vi "readWatchDog.vi"(8 "error in (no error)":errorcluster, 10 "id":T5=1, 11 "CoolerControler in":refnum<class "CoolerControler.lvclass">) -> (0 "error out":errorcluster, 1 "AS":T2, 2 "PS":T3, 3 "CoolerControler out":refnum<class "CoolerControler.lvclass">, 4 "WS":T1, 5 "CS":T4)   [LabVIEW 2016, in "CoolerControler.lvclass"]
uses:
  CoolerControler.lvclass
  typedefs/CoolerId.ctl
  typedefs/ControlStatusMode.ctl
  typedefs/PumpStatusFlag.ctl
  typedefs/AlarmStatusFlag.ctl
  typedefs/WarningStatusFlag.ctl
  typedefs/CoolerQuery.ctl
  SerialCommand/CoolerSerialCommand.lvclass
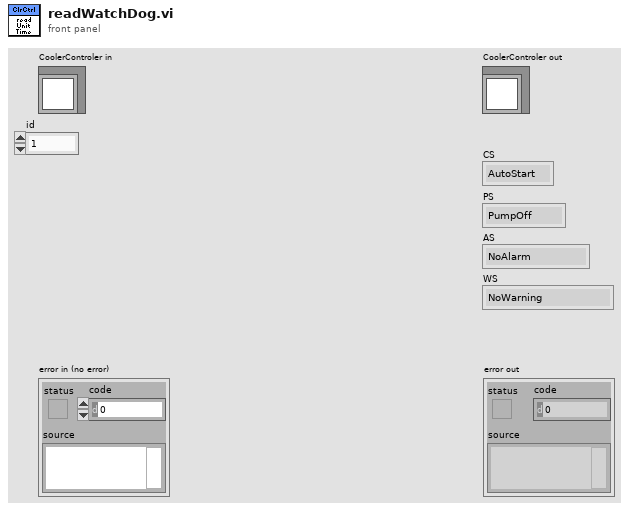
[diagram p1: front panel]
types:
  T1 = typedef "WarningStatusFlag.ctl" = enum16{"NoWarning", "WarningPresent"}
  T2 = typedef "AlarmStatusFlag.ctl" = enum16{"NoAlarm", "AlarmPresent"}
  T3 = typedef "PumpStatusFlag.ctl" = enum16{"PumpOff", "PumpOn"}
  T4 = typedef "ControlStatusMode.ctl" = enum16{"AutoStart", "Standby", "Run", "Safety", "Test"}
  T5 = typedef "CoolerId.ctl" = u16
  T6 = typedef "CoolerQuery.ctl" = enum16{"ReadSerialWatchdog", "ReadControlSensor", "ReadSetTemperature", "ReadSupplyTemperature", "ReadExternalRTD", "ReadExternalThermistor", "ReadReturnTemperature", "ReadAmbientTemperature", "ReadProcessFlow", "ReadTECBank1Current", "ReadTECBank2Current", "ReadTEDriveLevel", "ReadAlarmStateLevel1", "ReadAlarmStateLevel21", "ReadAlarmStateLevel22", "ReadWarningStateLevel1", "ReadHighSupplyTempWarning", "ReadLowSupplyTempWarning", "ReadHighAmbientTempWarning", "ReadLowAmbientTempWarning", "ReadLowProcessFlowWarning", "ReadHighSupplyTempAlarm", "ReadLowSupplyTempAlarm", "ReadHighAmbientTempAlarm", "ReadLowAmbientTempAlarm", "ReadLowProcessFlowAlarm", "ReadPWMandRelayStatus", "ReadPIDStatus", "ReadUnitUpTime", "ReadFan1Speed", "ReadFan2Speed", "ReadFan3Speed", "ReadFan4Speed"}
  T7 = typedef "response.ctl" = cluster{"deviceId":string, "commandNumber":string, "errorActive":bool, "commandName":string, "responseData":string, "checkSum":string}
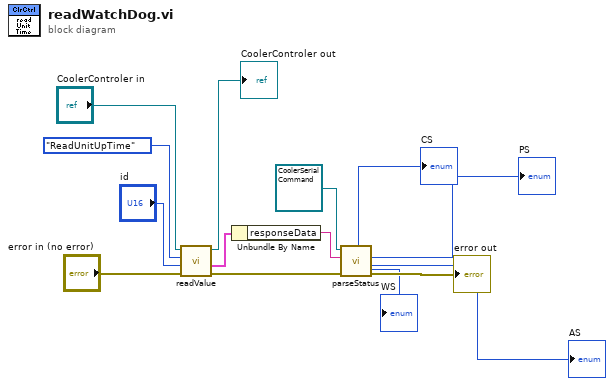
[diagram p0: block diagram]
diagram:
  n1 = call "readValue.vi"("error in (no error)"="error in (no error)", "id"="id", "CoolerQuery"=CoolerQuery."ReadUnitUpTime", "CoolerControler in"="CoolerControler in") -> ("error out"=w6:errorcluster, "response out"=w9:T7, "CoolerControler out"=→"CoolerControler out":refnum<class "CoolerControler.lvclass">)  [unwired: 4 in, 1 out]
  n2 = Unbundle By Name(w9) -> ("responseData"=w7:string)
  n3 = call "parseStatus.vi"("error in (no error)"=w6, "commandResponse"=w7, "CoolerSerialCommand in"=refnum<class "CoolerSerialCommand.lvclass"> refnum) -> ("error out"=→"error out":errorcluster, "AS"=→"AS":T2, "PS"=→"PS":T3, "WS"=→"WS":T1, "CS"=→"CS":T4)  [unwired: 3 in, 1 out]
